vi "PDC_SetColorTempMode.vi"(0 "DeviceNo":u32, 1 "R":u32, 2 "G":u32, 5 "ChildNo":u32, 7 "Mode":u32, 11 "error in (no error)":errorcluster, 12 "B":u32) -> (4 "ReturnValue":u32, 14 "ErrorCode":u32, 15 "error out":errorcluster)   [LabVIEW 2015]
doc: "This VI sets the color temperature status of the specified child device."
uses:
  PDCLIB.dll
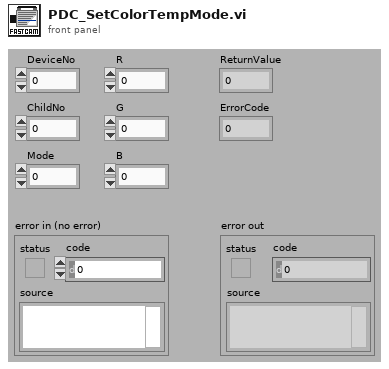
[diagram p1: front panel]
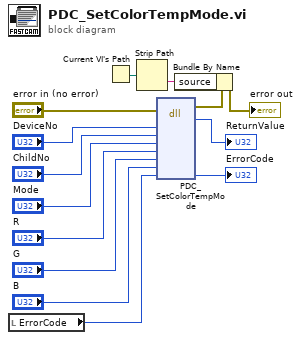
[diagram p0: block diagram]
diagram:
  n1 = local read "ErrorCode"() -> (w11:u32)
  n2 = Current VI's Path() -> (path=w3:path)
  n3 = Strip Path(path=w3) -> (name=w4:string)  [unwired: 1 out]
  n4 = dll-call lib="PDCLIB.dll" fn="PDC_SetColorTempMode"(error in="error in (no error)", "nDeviceNo"="DeviceNo", "nChildNo"="ChildNo", "nMode"="Mode", "nR"="R", "nG"="G", "nB"="B", "pErrorCode"=w11) -> (error out=w2:errorcluster, "return type"=→"ReturnValue":u32, "pErrorCode"=→"ErrorCode":u32)  [unwired: 8 in, 1 out]
  n5 = Bundle By Name(cluster=w2, "source"=w4) -> (→"error out":errorcluster)
